vi "Bias_adjustment.vi"(0 "Base current":dbl=1e-07 format="%#_6p", 1 "Two terminal IV":cluster{dbl[], dbl[]}(graph)={array[2480 elements], array[2480 elements]}, 2 "OSC Configuration":T1(array[cluster])=[{"Signal Type"=enum."Sine Wave", "DC"=0.006, "Amplitude"=0.025, "frequency"=1.0, "Phase"=0.0}, {"Signal Type"=enum."Sine Wave", "DC"=0.0, "Amplitude"=0.0, "frequency"=1.0, "Phase"=0.0}, {"Signal Type"=enum."Sine Wave", "DC"=0.0, "Amplitude"=0.0, "frequency"=1.0, "Phase"=0.0}, {"Signal Type"=enum."Sine Wave", "DC"=0.0, "Amplitude"=0.0, "frequency"=1.0, "Phase"=0.0}] {"frequency" format="%0.2p"; "Amplitude" format="%0.2p"; "DC" min=-0.99 max=0.99 format="%.2p"}, 3 "Delta":dbl=0.001) -> (5 "OSC Configuration 2":T1(array[cluster])=[{"Signal Type"=enum."Sine Wave", "DC"=0.006074066732632968, "Amplitude"=0.02298844279906127, "frequency"=1.0, "Phase"=0.0}, {"Signal Type"=enum."Sine Wave", "DC"=0.0, "Amplitude"=0.0, "frequency"=1.0, "Phase"=0.0}, {"Signal Type"=enum."Sine Wave", "DC"=0.0, "Amplitude"=0.0, "frequency"=1.0, "Phase"=0.0}, {"Signal Type"=enum."Sine Wave", "DC"=0.0, "Amplitude"=0.0, "frequency"=1.0, "Phase"=0.0}] {"frequency" format="%0.2p"; "Amplitude" format="%0.2p"; "DC" min=-0.99 max=0.99 format="%.2p"})   [LabVIEW 2016]
uses:
  <vilib>/gmath/NI_Gmath.lvlib
panel:
  out "Amp":dbl=0.02298844279906127
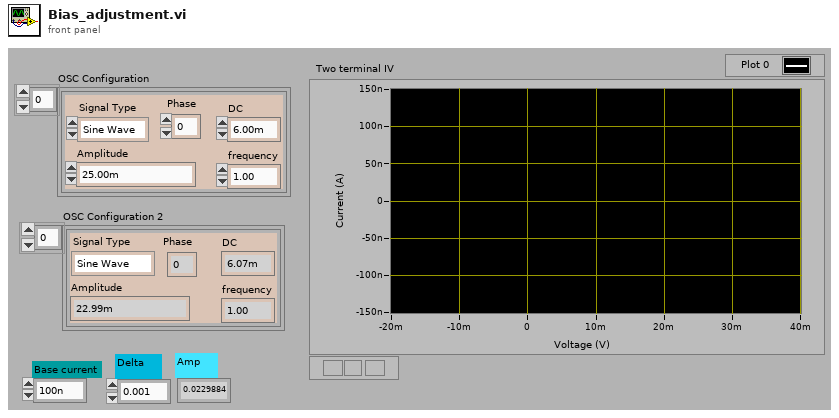
[diagram p1: front panel]
types:
  T1 = cluster{"Signal Type":enum16{"Sine Wave", "Triangle Wave", "Square Wave", "Sawtooth Wave"}, "DC":dbl, "Amplitude":dbl, "frequency":dbl, "Phase":dbl}[]
  T2 = cluster{"Signal Type":enum16{"Sine Wave", "Triangle Wave", "Square Wave", "Sawtooth Wave"}, "DC":dbl, "Amplitude":dbl, "frequency":dbl, "Phase":dbl}
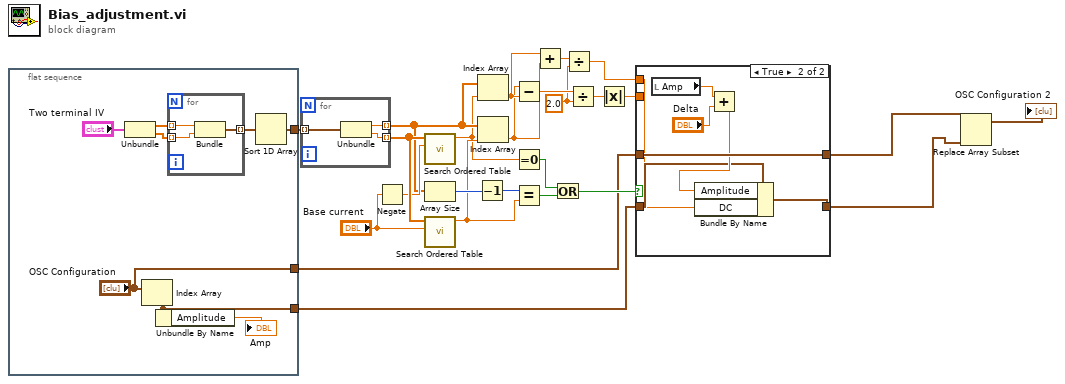
[diagram p0: block diagram]
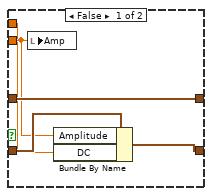
[diagram p2: hidden frame]
diagram:
  w3 = 2.0 ("y")
  n1 = flat-sequence {
    tunnel: [w31] -> w24
    tunnel: ["OSC Configuration"] -> w10
    tunnel: [w26] -> w9
    frame #0 {
      n2 = Unbundle("Two terminal IV") -> (w30:dbl[], w29:dbl[])
      n3 = Index Array(array="OSC Configuration") -> (element=w26:T2)  [unwired: 1 in]
      n4 = Unbundle By Name(w26) -> ("Amplitude"=→"Amp":dbl)
      n5 = for {
        tunnel: w30 -> [w36] mode=indexing
        tunnel: w29 -> [w35] mode=indexing
        tunnel: [w34] -> w32 mode=indexing
        n6 = Bundle(w36, w35) -> (w34:cluster{dbl, dbl})  [unwired: 1 in]
      }
      n7 = Sort 1D Array(array=w32) -> (sorted array=w31:cluster{dbl, dbl}[])
    }
  }
  n8 = for {
    tunnel: w24 -> [w39] mode=indexing
    tunnel: [w38] -> w23 mode=indexing
    tunnel: [w37] -> w18 mode=indexing
    n9 = Unbundle(w39) -> (w37:dbl, w38:dbl)
  }
  n10 = Negate(x="Base current") -> (-x=w20:dbl)
  n11 = call <vilib>:"Search Ordered Table.vi"("x value"=w20, "ordered x array"=w23) -> ("fractional index"=w11:dbl)  [unwired: 9 in]
  n12 = Array Size(array=w18) -> (size(s)=w17:i32)
  n13 = call <vilib>:"Search Ordered Table.vi"("x value"="Base current", "ordered x array"=w23) -> ("fractional index"=w12:dbl)  [unwired: 9 in]
  n14 = Decrement(x=w17) -> (x-1=w16:i32)
  n15 = Index Array(array=w18, index=w11) -> (element=w6:dbl)
  n16 = Index Array(array=w18, index=w12) -> (element=w5:dbl)
  n17 = Subtract(x=w5, y=w6) -> (x-y=w25:dbl)
  n18 = Equal To 0?(x=w11) -> (x = 0?=w15:bool)
  n19 = Equal?(x=w16, y=w12) -> (x = y?=w14:bool)
  n20 = Add(x=w6, y=w5) -> (x+y=w4:dbl)
  n21 = Or(x=w15, y=w14) -> (x .or. y?=w13:bool)
  n22 = Divide(x=w4, y=w3) -> (x/y=w2:dbl)
  n23 = Divide(x=w25, y=w3) -> (x/y=w22:dbl)
  n24 = Absolute Value(x=w22) -> (abs(x)=w19:dbl)
  n25 = case shown="True" w13 {
    tunnel: w19 -> [w42 _]
    tunnel: w10 -> [w44 w50]
    tunnel: [w44 w50] -> w8
    tunnel: w9 -> [w43 w48]
    tunnel: [w40 w47] -> w1
    tunnel: w2 -> [w41 w45]
    frame False {
      n26 = local write "Amp"(w42) -> ()
      n27 = Bundle By Name(cluster=w43, "Amplitude"=w42, "DC"=w41) -> (w40:T2)
    }
    frame True {
      n28 = local read "Amp"() -> (w46:dbl)
      n29 = Add(x=w46, y="Delta") -> (x+y=w49:dbl)
      n30 = Bundle By Name(cluster=w48, "Amplitude"=w49, "DC"=w45) -> (w47:T2)
    }
  }
  n31 = Replace Array Subset(array=w8, new element=w1) -> (→"OSC Configuration 2":T1)  [unwired: 1 in]
